vi "_FPGA_Driver_FastADC.vi"(8 "Clk_in":bool) -> (0 "Clk_out":bool, 2 "Output":i16)   [LabVIEW 2018]
uses:
  <vilib>/rvi/eio/common/nirviEmuTemplateMethod_errors.vi
  <vilib>/eio/EIONode/EIONode.xnode
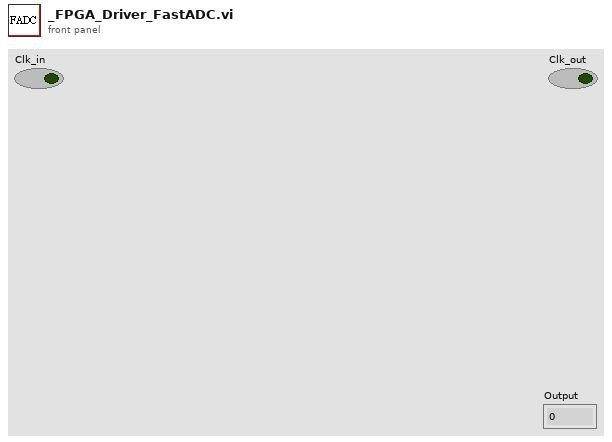
[diagram p1: front panel]
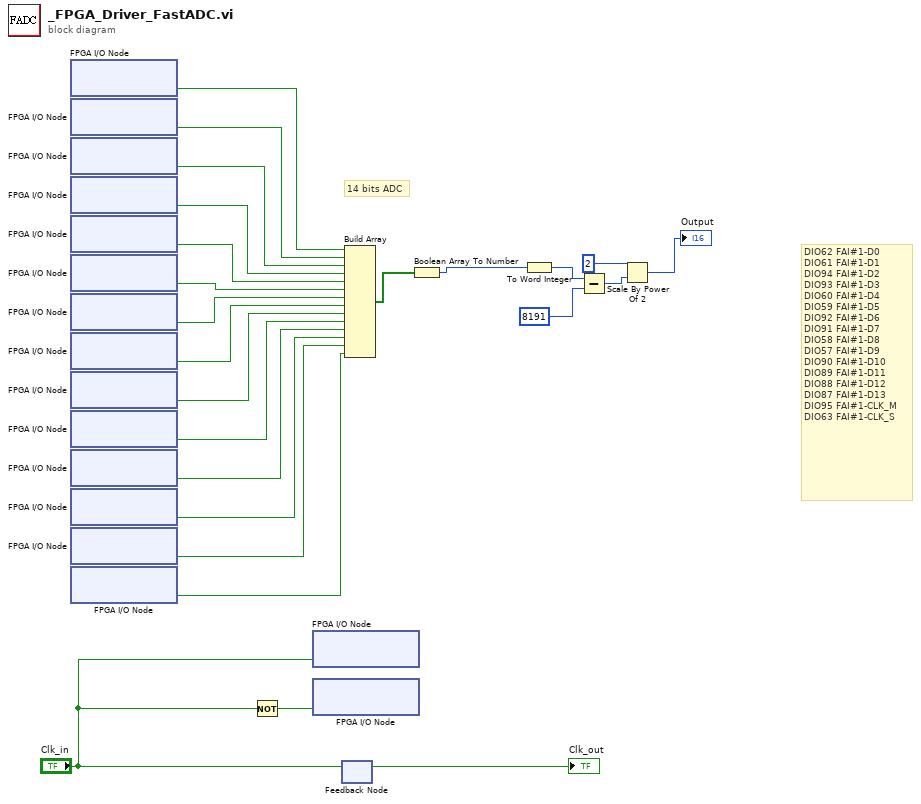
[diagram p0: block diagram]
diagram:
  # "14 bits ADC"
  # "DIO62\tFAI#1-D0\nDIO61\tFAI#1-D1\nDIO94\tFAI#1-D2\nDIO93\tFAI#1-D3\nDIO60\tFAI#1-D4\nDIO59\tFAI#1-D5\nDIO92\tFAI#1-D6\nDIO91\tFAI#1-D7\nDIO58\tFAI#1-D8\nDIO57\tFAI#1-D9\nDIO90\tFAI#1-D10\nDIO89\tFAI#1-D11\nDIO88\tFAI#1-D12\nDIO87\tFAI#1-D13\nDIO95\tFAI#1-CLK_M\nDIO63\tFAI#1-CLK_S"
  n1 = xnode "FPGA I/O Node"() -> ("RMC/DIO62"=w22:bool)  [unwired: 1 in, 1 out]
  n2 = xnode "FPGA I/O Node"() -> ("RMC/DIO61"=w21:bool)  [unwired: 1 in, 1 out]
  n3 = xnode "FPGA I/O Node"() -> ("RMC/DIO94"=w20:bool)  [unwired: 1 in, 1 out]
  n4 = xnode "FPGA I/O Node"() -> ("RMC/DIO93"=w19:bool)  [unwired: 1 in, 1 out]
  n5 = xnode "FPGA I/O Node"() -> ("RMC/DIO60"=w18:bool)  [unwired: 1 in, 1 out]
  n6 = xnode "FPGA I/O Node"() -> ("RMC/DIO59"=w17:bool)  [unwired: 1 in, 1 out]
  n7 = xnode "FPGA I/O Node"() -> ("RMC/DIO92"=w16:bool)  [unwired: 1 in, 1 out]
  n8 = xnode "FPGA I/O Node"() -> ("RMC/DIO91"=w15:bool)  [unwired: 1 in, 1 out]
  n9 = xnode "FPGA I/O Node"() -> ("RMC/DIO58"=w14:bool)  [unwired: 1 in, 1 out]
  n10 = xnode "FPGA I/O Node"() -> ("RMC/DIO57"=w13:bool)  [unwired: 1 in, 1 out]
  n11 = xnode "FPGA I/O Node"() -> ("RMC/DIO90"=w12:bool)  [unwired: 1 in, 1 out]
  n12 = xnode "FPGA I/O Node"() -> ("RMC/DIO89"=w11:bool)  [unwired: 1 in, 1 out]
  n13 = xnode "FPGA I/O Node"() -> ("RMC/DIO88"=w10:bool)  [unwired: 1 in, 1 out]
  n14 = xnode "FPGA I/O Node"() -> ("RMC/DIO87"=w9:bool)  [unwired: 1 in, 1 out]
  n15 = Not(x="Clk_in") -> (.not. x?=w7:bool)
  n16 = xnode "FPGA I/O Node"("RMC/DIO95"="Clk_in") -> ()  [unwired: 1 in, 1 out]
  n17 = xnode "FPGA I/O Node"("RMC/DIO63"=w7) -> ()  [unwired: 1 in, 1 out]
  n18 = feedback-in #1("Clk_in") -> ()
  n19 = feedback #1() -> (→"Clk_out":bool)  [unwired: 1 in]
  n20 = Build Array(w22, w21, w20, w19, w18, w17, w16, w15, w14, w13, w12, w11, w10, w9) -> (w8:bool[])
  n21 = Boolean Array To Number(Boolean array=w8) -> (number=w2:u16)
  n22 = To Word Integer(number=w2) -> (16bit integer=w24:i16)
  n23 = Subtract(x=w24, y=i16 8191) -> (x-y=w5:i16)
  n24 = Scale By Power Of 2(n=i16 2, x=w5) -> (x*2^n=→"Output":i16)
